vi "Ground_Station.vi"() -> ()   [LabVIEW 2018]
uses:
  hdlc/data_frame_types/frame_data_type.ctl
  hdlc/data_frame_types/data_pkg_t.ctl
  hdlc/data_frame_types/gps_data_t.ctl
  2213985a-ce5c-4bbe-9663-3d2ea05cd94b.vi
  eafdd0cf-07df-426f-9b74-3c0edbf6e6c1.vi
  3eaf0637-73f7-436c-9673-51bf41f0c9f4.vi
  0f17ee01-5a13-48db-ae0f-6ca45ead56a9.vi
  95fef445-3850-4ef1-ba1c-405eff07cc5a.vi
  8f023bd5-54de-4fa5-8c9e-7e05942e9f56.vi
  92fbc625-f3f8-423f-b0ed-2ece32d19a34.vi
  9502c997-2099-45ec-ac65-0f2f0cc1ee03.vi
  9d935f80-5509-49da-90a4-9453c0765d51.vi
  2de26032-b61c-4b53-b4f6-e587d9a9aaf6.vi
  e8886ea6-91be-41e7-bc4a-7c115d0a2f3e.vi
  041cc2b0-ec36-4d56-96d2-fee5723584a4.vi
  5810dd3f-7f00-499c-8001-2bb35bdbaa32.vi
  324ca73f-0aa5-43f7-a6ae-8032262acc61.vi
  38db9fbf-4e2c-458f-a3f4-03dcc44cfe3c.vi
  5ce1995e-e115-49f6-a00a-c996211abfd2.vi
  <vilib>/Instr/_visa.llb/VISA Configure Serial Port (Instr).vi
panel:
  in  "ADC Readings":T1(tab)
  out "ADC Channel 0":u16(graph)
  out "ADC Channel 1":u16(graph)
  out "ADC Channel 2":u16(graph)
  out "ADC Channel 3":u16(graph)
  out "ADC Channel 4":u16(graph)
  out "ADC Channel 5":u16(graph)
  out "ADC Channel 6":u16(graph)
  out "ADC Channel 7":u16(graph)
  out "accel_z":sgl
  out "accel_y":sgl
  out "accel_x":sgl
  out "angle_z":sgl
  out "angle_y":sgl
  out "angle_x":sgl
  out "sat_num":u8
  out "fix_qual":u8
  out "fix":bool
  out "lon":sgl format="%#.6f"
  out "lat":sgl format="%.6f"
  out "sec":u8
  out "min":u8
  out "hour":u8
  out "day":u8
  out "month":u8
  out "year":u8
  out "ADC_0":u16(knob) scale=0.0..1023.0
  in  "New upper limit":u8
  out "Rand Data":u8(graph)
  in  "stop":bool
  in  "Send":bool
  in  "VISA resource name":refnum<visa-resource-name>
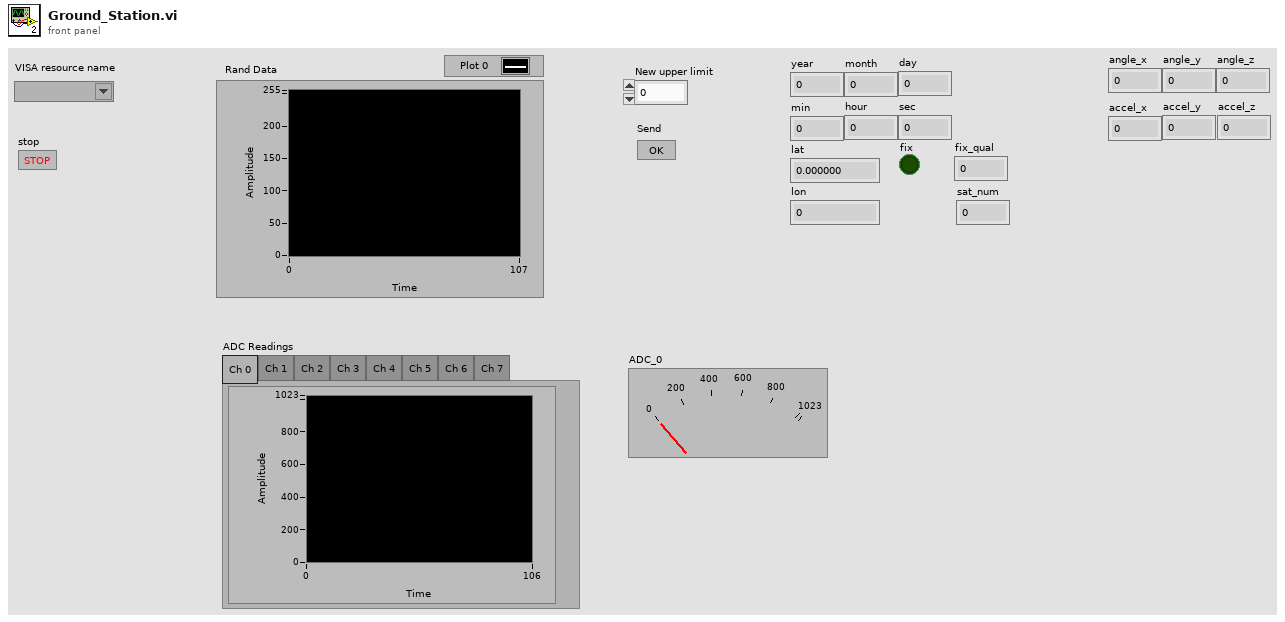
[diagram p1: front panel]
types:
  T1 = enum32{"Ch 0", "Ch 1", "Ch 2", "Ch 3", "Ch 4", "Ch 5", "Ch 6", "Ch 7"}
  T2 = typedef "frame_data_type.ctl" = enum8{"SENSOR_DATA", "RND_MAX", "GPS_DATA"}
  T3 = typedef "data_pkg_t.ctl" = cluster{"rand_num":u8, "adc_chnl_0":u16, "adc_chnl_1":u16, "adc_chnl_2":u16, "adc_chnl_3":u16, "adc_chnl_4":u16, "adc_chnl_5":u16, "adc_chnl_6":u16, "adc_chnl_7":u16, "angle_x":sgl, "angle_y":sgl, "angle_z":sgl, "accel_x":sgl, "accel_y":sgl, "accel_z":sgl}
  T4 = typedef "gps_data_t.ctl" = cluster{"year":u8, "month":u8, "day":u8, "hour":u8, "min":u8, "sec":u8, "lat":sgl, "lon":sgl, "fix":bool, "fix_qual":u8, "sat_num":u8}
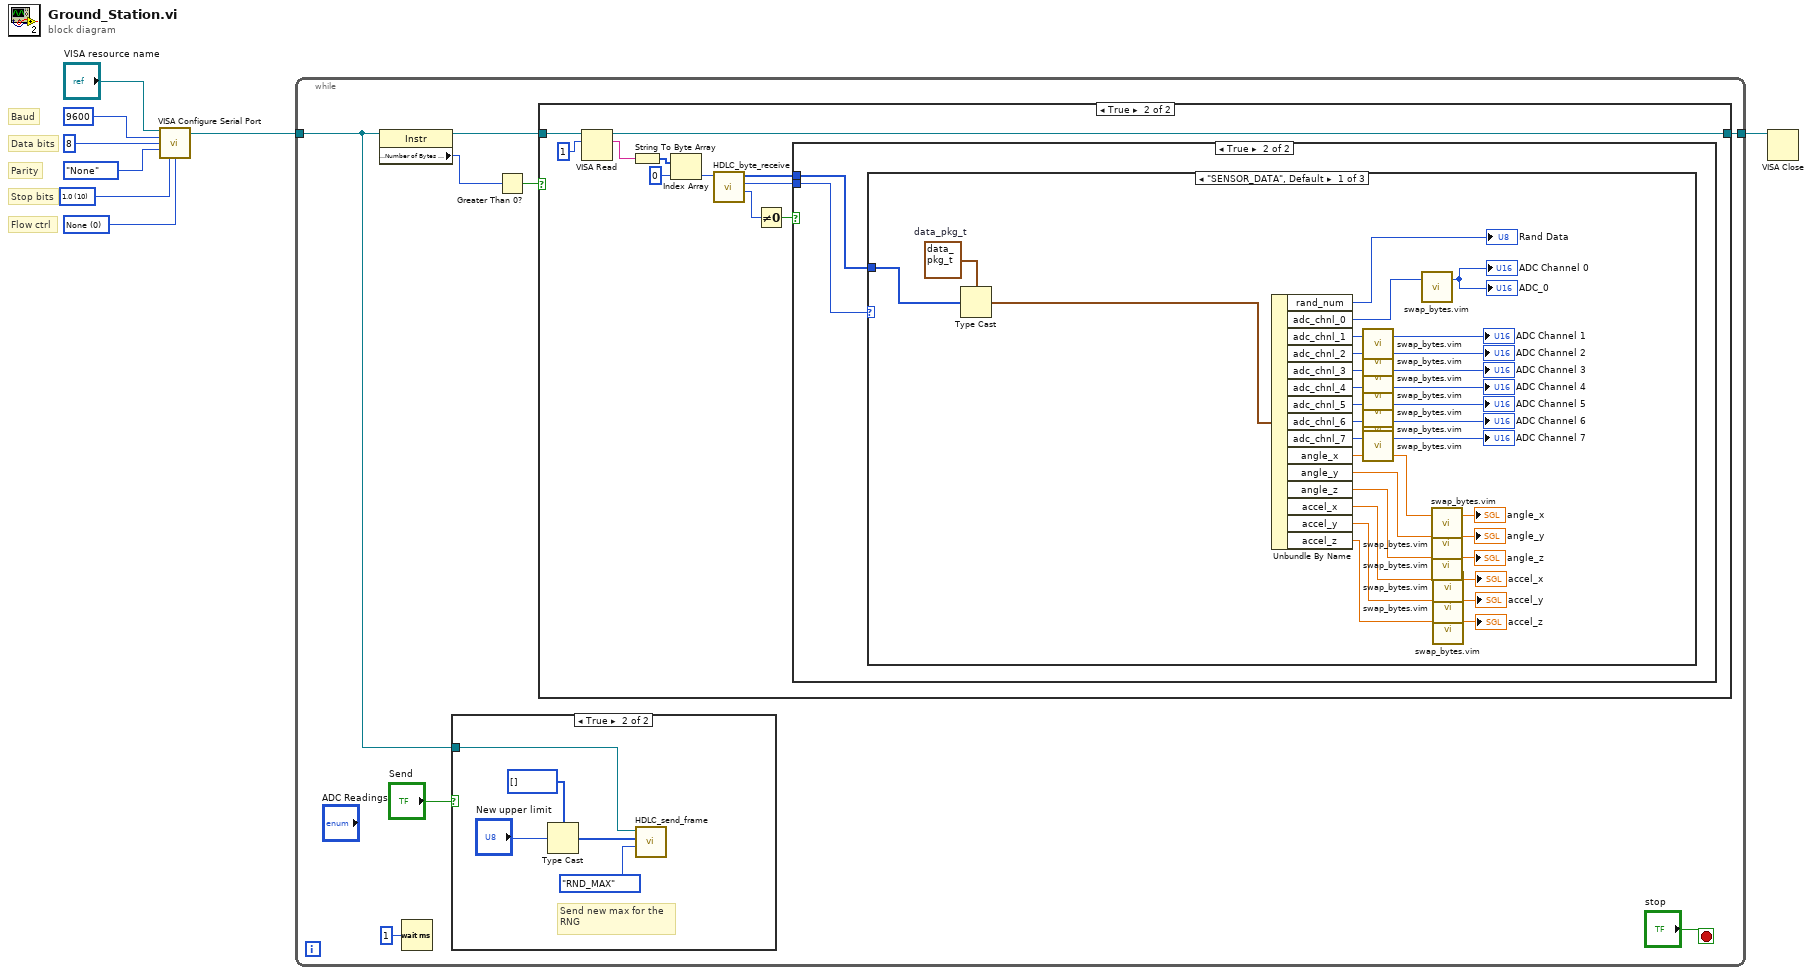
[diagram p0: block diagram]
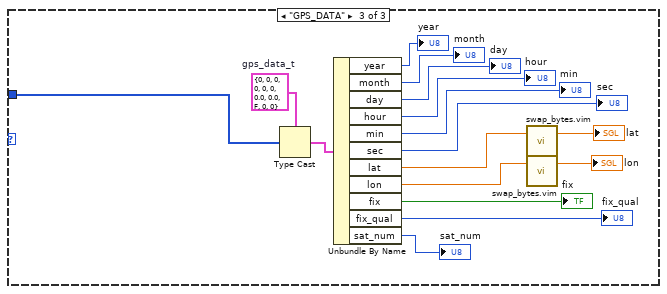
[diagram p5: hidden frame]
diagram:
  w3 = u16 0 items=["None", "XON/XOFF", "RTS/CTS", "XON/XOFF & RTS/CTS", "DTR/DSR", "XON/XOFF & DTR/DSR"] ("flow control (0:none)")
  w4 = u16 10 items=["1.0"=10, "1.5"=15, "2.0"=20] ("stop bits (10: 1 bit)")
  # "Flow ctrl"
  # "Stop bits"
  # "Parity"
  # "Data bits"
  # "Baud"
  n1 = call-poly "VISA Configure Serial Port"("VISA resource name"="VISA resource name", "baud rate (9600)"=u32 9600, "data bits (8)"=u16 8, "parity (0:none)"=enum16{"None", "Odd", "Even", "Mark", "Space"}."None", "stop bits (10: 1 bit)"=w4, "flow control (0:none)"=w3) -> ("VISA resource name out"=w2:refnum<visa-resource-name>)  [unwired: 8 in, 1 out]
  n2 = while {
    tunnel: w2 -> [w12]
    tunnel: [w15] -> w1
    stop <- "stop" stop-if-true
    n3 = property class="Instr"(reference=w12) -> (reference out=w16:refnum<visa-resource-name>, "Serial Settings:Number of Bytes at Serial Port"=w10:u32)  [unwired: 1 in, 1 out]
    n4 = Wait (ms)(milliseconds to wait=u32 1) -> ()  [unwired: 1 out]
    n5 = case shown="True" "Send" {
      tunnel: w12 -> [_ w81]
      frame False {
      }
      frame True {
        # "Send new max for the\nRNG"
        n6 = Type Cast(type=u8[] [], x="New upper limit") -> (*(type *) &x=w80:u8[])
        n7 = call "HDLC_send_frame.vi"("data_type"=frame_data_type."RND_MAX", "data"=w80, "VISA resource name"=w81) -> ()  [unwired: 9 in]
      }
    }
    n8 = Greater Than 0?(x=w10) -> (x > 0?=w11:bool)
    n9 = case shown="True" w11 {
      tunnel: w16 -> [w17 w28]
      tunnel: [w17 w27] -> w15
      frame False {
      }
      frame True {
        n10 = VISA Read(VISA resource name=w28, byte count=u32 1) -> (VISA resource name out=w27:refnum<visa-resource-name>, read buffer=w25:string)  [unwired: 1 in, 2 out]
        n11 = String To Byte Array(string=w25) -> (unsigned byte array=w24:u8[])
        n12 = Index Array(array=w24, index=0) -> (element=w22:u8)
        n13 = call "HDLC_byte_receive.vi"("new_byte"=w22) -> ("frame_size"=w20:u8, "data_type"=w18:T2, "frame"=w19:u8[])  [unwired: 7 in]
        n14 = Not Equal To 0?(x=w20) -> (x != 0?=w21:bool)
        n15 = case shown="True" w21 {
          tunnel: w19 -> [_ w30]
          tunnel: w18 -> [_ w29]
          frame False {
          }
          frame True {
            n16 = case shown="\"SENSOR_DATA\", Default" w29 {
              tunnel: w30 -> [w59 _ w68]
              frame "SENSOR_DATA", Default {
                w60 = T3 {"rand_num"=0, "adc_chnl_0"=0, "adc_chnl_1"=0, "adc_chnl_2"=0, "adc_chnl_3"=0, "adc_chnl_4"=0, "adc_chnl_5"=0, "adc_chnl_6"=0, "adc_chnl_7"=0, "angle_x"=0.0, "angle_y"=0.0, "angle_z"=0.0, "accel_x"=0.0, "accel_y"=0.0, "accel_z"=0.0}  # data_pkg_t
                n17 = Type Cast(type=w60, x=w59) -> (*(type *) &x=w62:T3)
                n18 = Unbundle By Name(w62) -> ("rand_num"=→"Rand Data":u8, "adc_chnl_0"=w52:u16, "adc_chnl_1"=w38:u16, "adc_chnl_2"=w39:u16, "adc_chnl_3"=w40:u16, "adc_chnl_4"=w41:u16, "adc_chnl_5"=w42:u16, "adc_chnl_6"=w43:u16, "adc_chnl_7"=w44:u16, "angle_x"=w58:sgl, "angle_y"=w56:sgl, "angle_z"=w55:sgl, "accel_x"=w47:sgl, "accel_y"=w46:sgl, "accel_z"=w45:sgl)
                n19 = call "swap_bytes.vim"("data"=w38) -> ("reversed"=→"ADC Channel 1":u16)  [unwired: 2 in]
                n20 = call "swap_bytes.vim"("data"=w39) -> ("reversed"=→"ADC Channel 2":u16)  [unwired: 2 in]
                n21 = call "swap_bytes.vim"("data"=w40) -> ("reversed"=→"ADC Channel 3":u16)  [unwired: 2 in]
                n22 = call "swap_bytes.vim"("data"=w41) -> ("reversed"=→"ADC Channel 4":u16)  [unwired: 2 in]
                n23 = call "swap_bytes.vim"("data"=w42) -> ("reversed"=→"ADC Channel 5":u16)  [unwired: 2 in]
                n24 = call "swap_bytes.vim"("data"=w43) -> ("reversed"=→"ADC Channel 6":u16)  [unwired: 2 in]
                n25 = call "swap_bytes.vim"("data"=w44) -> ("reversed"=→"ADC Channel 7":u16)  [unwired: 2 in]
                n26 = call "swap_bytes.vim"("data"=w52) -> ("reversed"=→"ADC Channel 0" →"ADC_0":u16)  [unwired: 2 in]
                n27 = call "swap_bytes.vim"("data"=w58) -> ("reversed"=→"angle_x":sgl)  [unwired: 2 in]
                n28 = call "swap_bytes.vim"("data"=w56) -> ("reversed"=→"angle_y":sgl)  [unwired: 2 in]
                n29 = call "swap_bytes.vim"("data"=w55) -> ("reversed"=→"angle_z":sgl)  [unwired: 2 in]
                n30 = call "swap_bytes.vim"("data"=w47) -> ("reversed"=→"accel_x":sgl)  [unwired: 2 in]
                n31 = call "swap_bytes.vim"("data"=w46) -> ("reversed"=→"accel_y":sgl)  [unwired: 2 in]
                n32 = call "swap_bytes.vim"("data"=w45) -> ("reversed"=→"accel_z":sgl)  [unwired: 2 in]
              }
              frame "RND_MAX" {
                # "Only used for sending data"
              }
              frame "GPS_DATA" {
                w78 = T4 {"year"=0, "month"=0, "day"=0, "hour"=0, "min"=0, "sec"=0, "lat"=0.0, "lon"=0.0, "fix"=FALSE, "fix_qual"=0, "sat_num"=0}  # gps_data_t
                n33 = Type Cast(type=w78, x=w68) -> (*(type *) &x=w77:T4)
                n34 = Unbundle By Name(w77) -> ("year"=→"year":u8, "month"=→"month":u8, "day"=→"day":u8, "hour"=→"hour":u8, "min"=→"min":u8, "sec"=→"sec":u8, "lat"=w66:sgl, "lon"=w64:sgl, "fix"=→"fix":bool, "fix_qual"=→"fix_qual":u8, "sat_num"=→"sat_num":u8)
                n35 = call "swap_bytes.vim"("data"=w66) -> ("reversed"=→"lat":sgl)  [unwired: 2 in]
                n36 = call "swap_bytes.vim"("data"=w64) -> ("reversed"=→"lon":sgl)  [unwired: 2 in]
              }
            }
          }
        }
      }
    }
  }
  n37 = VISA Close(VISA resource name=w1) -> ()  [unwired: 1 in, 1 out]
